vi "Filter Panel.vi"(5 "Col":i32, 7 "Row":i32, 8 "error in (no error)":errorcluster, 10 "Panel":refnum<class "ArrayPanel.lvclass">, 11 "Panel Filter in":refnum<class "Panel Filter.lvclass">) -> (0 "error out":errorcluster, 2 "Include":bool, 3 "Panel Filter out":refnum<class "Panel Filter.lvclass">)   [LabVIEW 2020, in "OOPanel.lvlib" / "Panel Filter.lvclass"]
uses:
  Panel Filter.lvclass
  ArrayPanel/ArrayPanel.lvclass
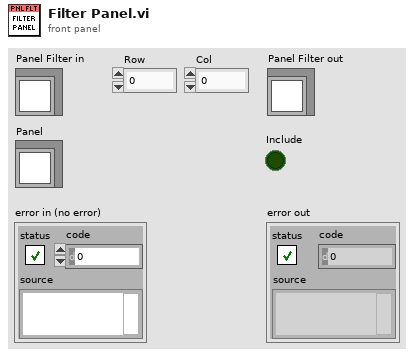
[diagram p1: front panel]
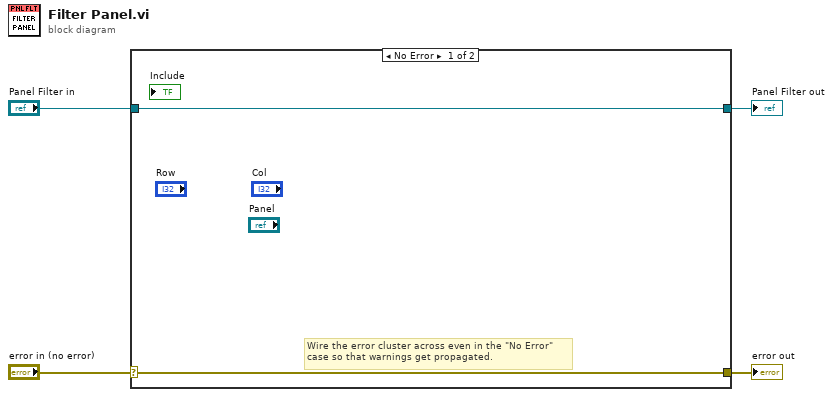
[diagram p0: block diagram]
diagram:
  n1 = case shown="No Error" "error in (no error)" {
    selector: "error in (no error)" -> [w5 w8]
    tunnel: [w5 w8] -> w3
    tunnel: [w6 w7] -> w1
    tunnel: "Panel Filter in" -> [w6 w7]
    frame No Error {
      # "Wire the error cluster across even in the \"No Error\"\ncase so that warnings get propagated."
    }
    frame Error {
    }
  }
  "error out" <- w3
  "Panel Filter out" <- w1
